vi "Write Step State.vi"(8 "error in (no error)":errorcluster, 10 "Step State":T1={"Result"="N/A", "Status"="IDLE", "Enabled"=TRUE, "Upper"="", "Target"="", "Lower"="", "Value"=""}, 11 "Base Step in":refnum<class "Base Step.lvclass">) -> (0 "error out":errorcluster, 3 "Base Step out":refnum<class "Base Step.lvclass">)   [LabVIEW 2024, in "Ramses Sequencer.lvlib" / "Base Step.lvclass"]
uses:
  Base Step.lvclass
  Typedefs/Step State.ctl
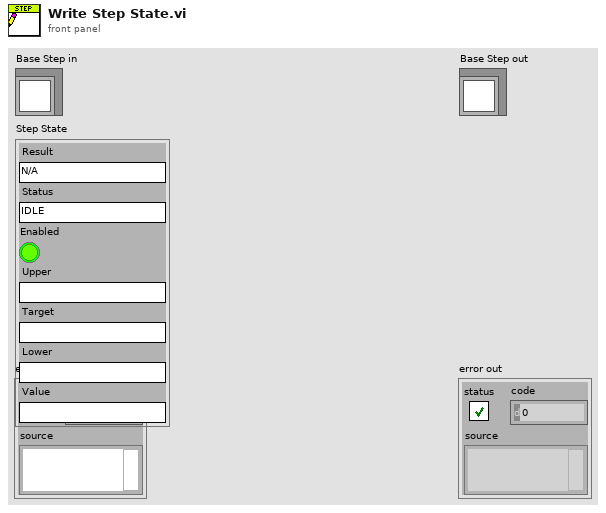
[diagram p1: front panel]
types:
  T1 = typedef "Ramses Sequencer.lvlib/Base Step.lvclass/Step State.ctl" = cluster{"Result":string, "Status":string, "Enabled":bool, "Upper":string, "Target":string, "Lower":string, "Value":string}
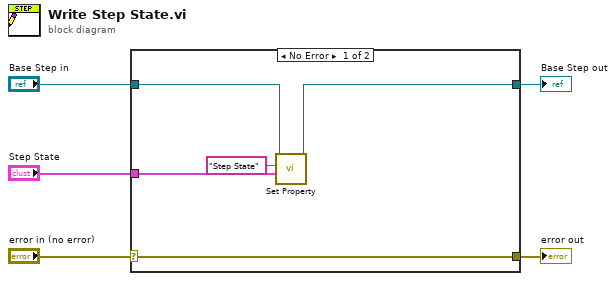
[diagram p0: block diagram]
diagram:
  n1 = case shown="No Error" "error in (no error)" {
    selector: "error in (no error)" -> [w10 w11]
    tunnel: [w10 w11] -> w4
    tunnel: [w9 w12] -> w2
    tunnel: "Base Step in" -> [w8 w12]
    tunnel: "Step State" -> [w7 _]
    frame No Error {
      n2 = call "Set Property.vi"("Data"=w7, "Key"="Step State", "Base Step in"=w8) -> ("Base Step out"=w9:refnum<class "Base Step.lvclass">)  [unwired: 7 in, 1 out]
    }
    frame Error {
    }
  }
  "error out" <- w4
  "Base Step out" <- w2
